vi "optogeneticsExecuteIntervalScan.vi"() -> ()   [LabVIEW 2017]
uses:
  globalDevices.vi
  globalUtilities.vi
panel:
  out "elapsed time (s)":dbl format="%#2.1g"
  out "currentTimeBtwTrains (s)":dbl
  in  "nTrains":i32=2
  in  "timeBtwTrains (s)":dbl[](array[numeric])=[0.0]
  out "pharosFire":bool
  in  "executeStep":bool
  in  "stimulus duration (s)":dbl=1.0
  in  "repRateDivider":i32=1
  out "nPulses":i32
  # "SCAN IN DELAY BETWEEN TWO TRAINS OF PULSES\nEnable external control in pharosControl.\nUse the appropriate software for spatial targeting. This VI only deals with the laser pulses."
  # "SET"
  # "DIAGNOSTICS"
  # "EXECUTE STEP AND FIRE LASER PULSES"
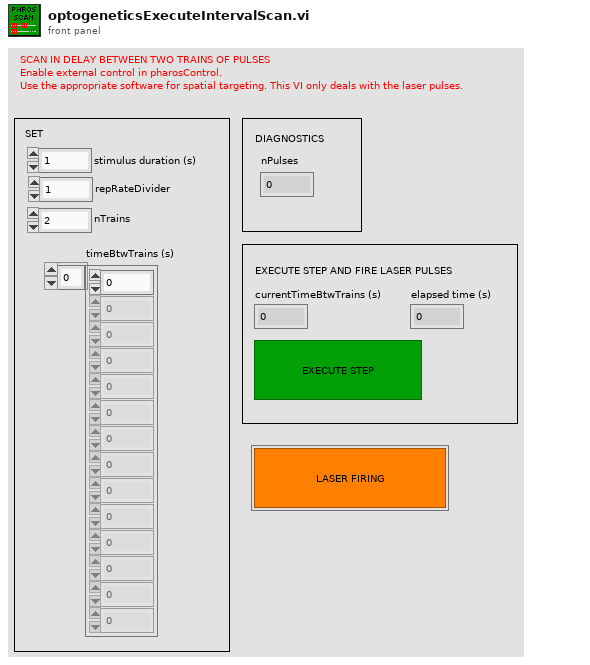
[diagram p1: front panel]
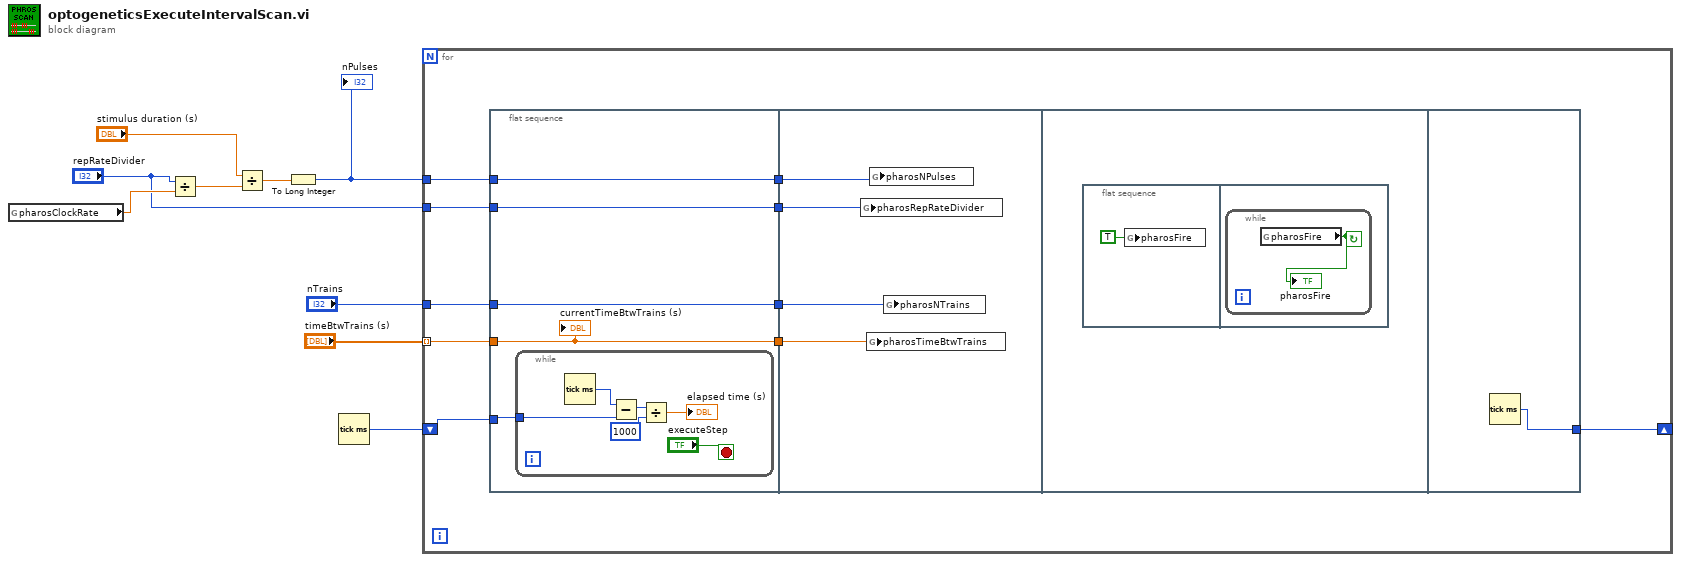
[diagram p0: block diagram]
diagram:
  n1 = global read "globalDevices.vi" "pharosClockRate"() -> (w9:dbl)
  n2 = Divide(x="repRateDivider", y=w9) -> (x/y=w7:dbl)
  n3 = Divide(x="stimulus duration (s)", y=w7) -> (x/y=w6:dbl)
  n4 = To Long Integer(number=w6) -> (32bit integer=w5:i32)
  "nPulses" <- w5
  n5 = Tick Count (ms)() -> (millisecond timer value=w1:u32)
  n6 = for {
    tunnel: w5 -> [w18]
    tunnel: "repRateDivider" -> [w16]
    tunnel: "timeBtwTrains (s)" -> [w14] mode=indexing
    tunnel: "nTrains" -> [w13]
    shift-right: [w10] -> _
    shift-left: w1 -> [w11]
    n7 = flat-sequence {
      tunnel: [w24] -> w19
      tunnel: w18 -> [w24]
      tunnel: [w23] -> w17
      tunnel: w16 -> [w23]
      tunnel: [w22] -> w15
      tunnel: w14 -> [w22]
      tunnel: w13 -> [w21]
      tunnel: [w21] -> w12
      tunnel: w11 -> [w20]
      tunnel: w19 -> [w34]
      tunnel: w17 -> [w33]
      tunnel: w15 -> [w32]
      tunnel: w12 -> [w31]
      tunnel: [w37] -> w10
      frame #0 {
        n8 = while {
          tunnel: w20 -> [w25]
          stop <- "executeStep" stop-if-true
          n9 = Tick Count (ms)() -> (millisecond timer value=w29:u32)
          n10 = Subtract(x=w29, y=w25) -> (x-y=w28:u32)
          n11 = Divide(x=w28, y=u32 1000) -> (x/y=→"elapsed time (s)":dbl)
        }
        "currentTimeBtwTrains (s)" <- w22
      }
      frame #1 {
        n12 = global write "globalUtilities.vi" "pharosRepRateDivider"(w33) -> ()
        n13 = global write "globalUtilities.vi" "pharosTimeBtwTrains"(w32) -> ()
        n14 = global write "globalUtilities.vi" "pharosNPulses"(w34) -> ()
        n15 = global write "globalUtilities.vi" "pharosNTrains"(w31) -> ()
      }
      frame #2 {
        n16 = flat-sequence {
          frame #0 {
            n17 = global write "globalUtilities.vi" "pharosFire"(TRUE ("pharosFire")) -> ()
          }
          frame #1 {
            n18 = while {
              stop <- w36 continue-if-true
              n19 = global read "globalUtilities.vi" "pharosFire"() -> (w36:bool)
              "pharosFire" <- w36
            }
          }
        }
      }
      frame #3 {
        n20 = Tick Count (ms)() -> (millisecond timer value=w37:u32)
      }
    }
  }
